vi "Test 4.vi"(8 "error in (no error)":errorcluster, 11 "Test Case In":refnum<class "Tests Rev3.lvclass">) -> (0 "error out":errorcluster, 3 "Test Case Out":refnum<class "Tests Rev3.lvclass">)   [LabVIEW 2021, in "Tests Rev3.lvclass"]
uses:
  Tests Rev3.lvclass
  C:/Program Files (x86)/National Instruments/LabVIEW 2021/vi.lib/Astemes/LUnit/Test Case.lvclass
  <vilib>/Astemes/LUnit/Test Case.lvclass/Test Case.ctl
  4993e8ee-a06a-463a-9684-69129f64d5ce.vi
  <vilib>/Astemes/LUnit/Append Pass Result.vi
  <vilib>/Astemes/LUnit/Append Fail Result.vi
  <vilib>/Astemes/LUnit/Describe Comparison.vi
  <vilib>/Astemes/LUnit/Compare Variants.vi
  <vilib>/Astemes/LUnit/Variant to string.vi
  <vilib>/Utility/Data Type/Get Type Information.vi
  <vilib>/Utility/LVClass/Get LV Class Name.vi
  Proto/Group.lvclass
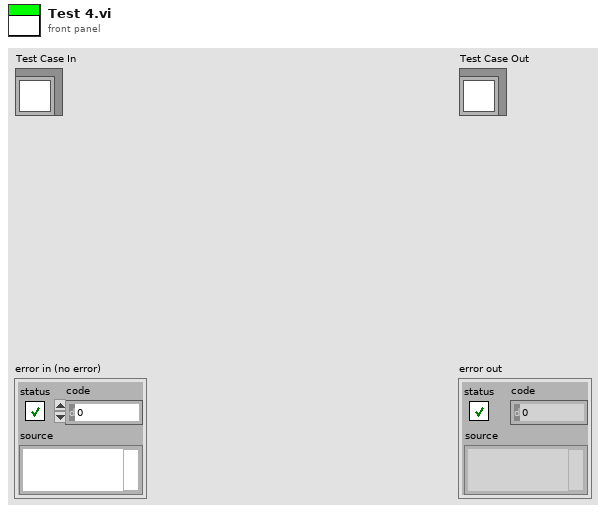
[diagram p1: front panel]
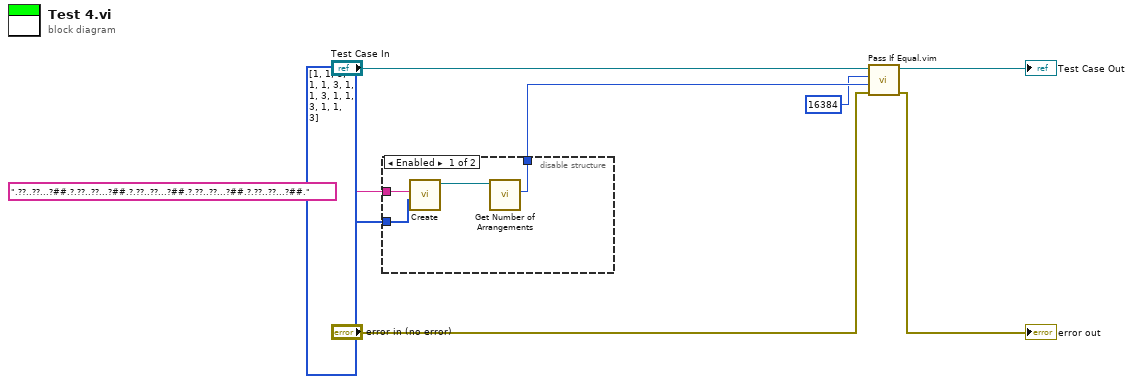
[diagram p0: block diagram]
diagram:
  n1 = disable-structure shown="Enabled" {
    disable-tunnel: ".??..??...?##.?.??..??...?##.?.??..??...?##.?.??..??...?##.?.??..??...?##." ("Input") -> [w12 _]
    disable-tunnel: [w10 _] -> w3
    disable-tunnel: i64[] [1, 1, 3, 1, 1, 3, 1, 1, 3, 1, 1, 3, 1, 1, 3] ("Group Sizes") -> [w9 _]
    frame Enabled {
      n2 = call "Create.vi"("Group Sizes"=w9, "Input"=w12) -> ("Group Out"=w11:refnum<class "Group.lvclass">)  [unwired: 8 in, 1 out]
      n3 = call "Get Number of Arrangements.vi"("Proto in"=w11) -> ("Arrangements"=w10:u64)  [unwired: 8 in, 2 out]
    }
    frame Disabled {
    }
  }
  n4 = call "Pass If Equal.vim"("error in (no error)"="error in (no error)", "Actual"=w3, "Expected"=u64 16384 ("Arrangements"), "LUnit Test Case In"="Test Case In") -> ("error out"=→"error out":errorcluster, "LUnit Test Case Out"=→"Test Case Out":refnum<class "Tests Rev3.lvclass">)  [unwired: 6 in]
